vi "shape0.vi"() -> ()   [LabVIEW 2020]
uses:
  bee2abb7-c490-4ad6-bfc0-30ed72578e14.vi
panel:
  out "Array":cluster{"x":dbl, "y":dbl}[](array[cluster])
  in  "input variable":dbl=5.5 format="%#_13g"
  out "XY Graph":cluster{dbl[], dbl[]}(graph)
  # "e"
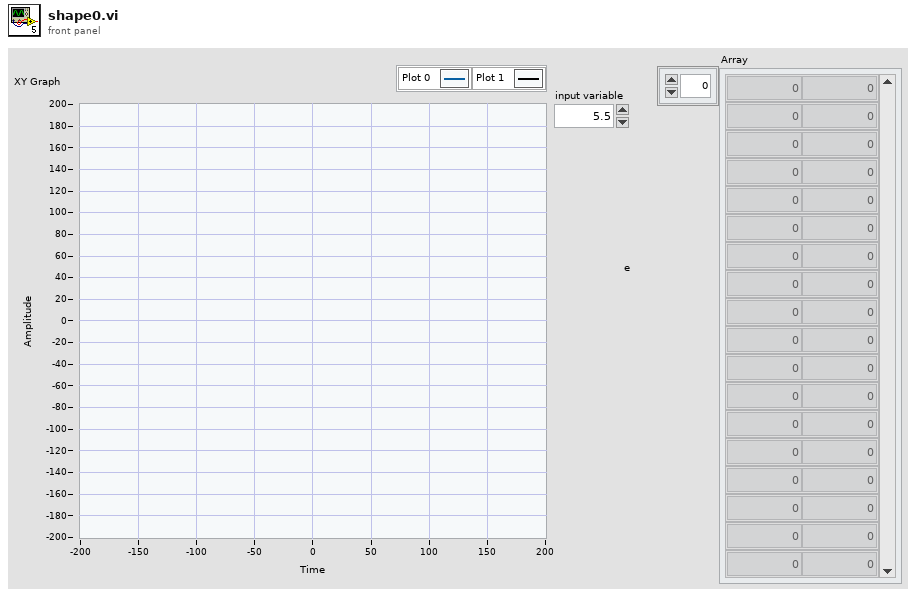
[diagram p1: front panel]
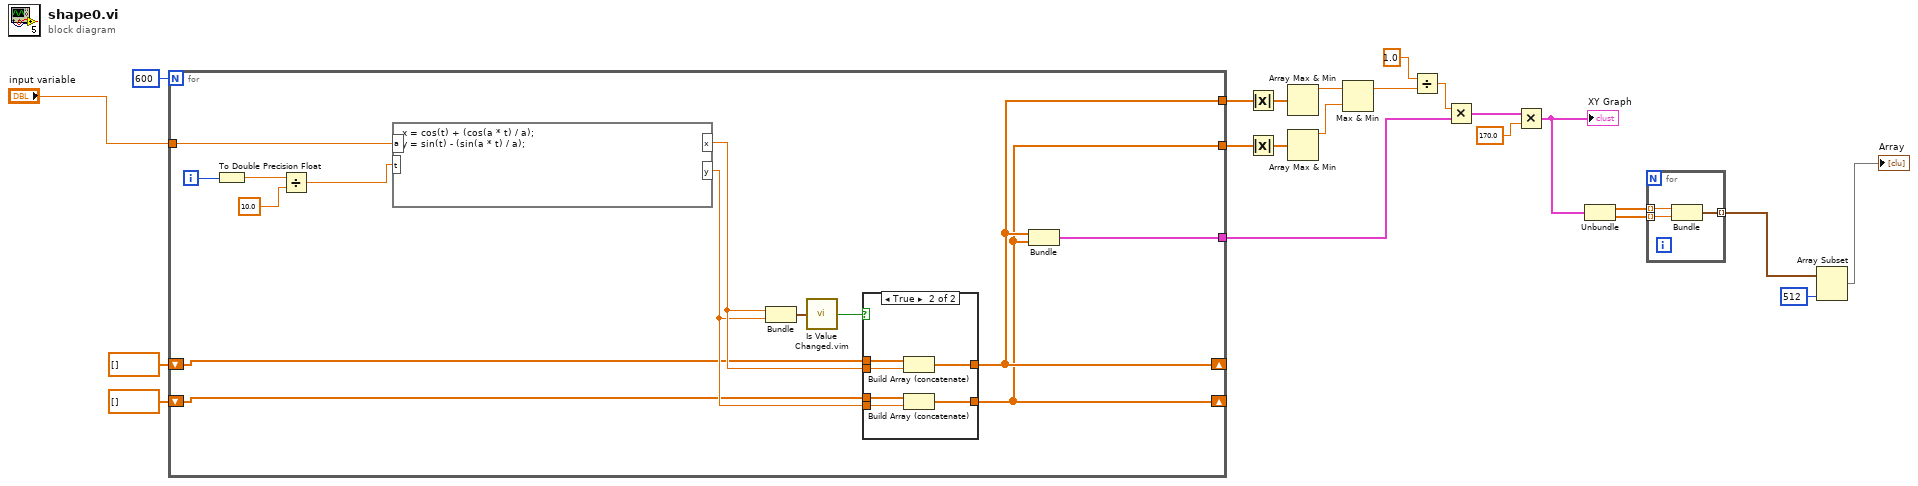
[diagram p0: block diagram]
diagram:
  n1 = for {
    N: 600 -> [_]
    tunnel: "input variable" -> [w36]
    shift-right: [w24] -> _
    shift-left: dbl[] [] -> [w31]
    shift-right: [w23] -> _
    shift-left: dbl[] [] -> [w30]
    tunnel: [w29] -> w9
    tunnel: [w24] -> w18
    tunnel: [w23] -> w17
    i -> [w28]
    n2 = To Double Precision Float(number=w28) -> (double precision float=w27:dbl)
    n3 = Divide(x=w27, y=10.0) -> (x/y=w25:dbl)
    n4 = formula code="x = cos(t) + (cos(a * t) / a);\ny = sin(t) - (sin(a * t) / a);"("a"=w36, "t"=w25) -> ("x"=w33:dbl, "y"=w32:dbl)
    n5 = Bundle("x"=w33, "y"=w32) -> (w35:cluster{"x":dbl, "y":dbl})  [unwired: 1 in]
    n6 = call "Is Value Changed.vim"("value"=w35) -> ("changed or first call?"=w34:bool)
    n7 = case shown="True" w34 {
      tunnel: w33 -> [_ w44]
      tunnel: w32 -> [_ w43]
      tunnel: [w38 w42] -> w24
      tunnel: [w37 w41] -> w23
      tunnel: w31 -> [w38 w40]
      tunnel: w30 -> [w37 w39]
      frame False {
      }
      frame True {
        n8 = Build Array (concatenate)(w40, w44) -> (w42:dbl[])
        n9 = Build Array (concatenate)(w39, w43) -> (w41:dbl[])
      }
    }
    n10 = Bundle(w24, w23) -> (w29:cluster{dbl[], dbl[]})  [unwired: 1 in]
  }
  n11 = Absolute Value(x=w18) -> (abs(x)=w16:dbl[])
  n12 = Absolute Value(x=w17) -> (abs(x)=w15:dbl[])
  n13 = Array Max & Min(array=w16) -> (max value=w14:dbl)  [unwired: 3 out]
  n14 = Array Max & Min(array=w15) -> (max value=w13:dbl)  [unwired: 3 out]
  n15 = Max & Min(x=w14, y=w13) -> (max(x,y)=w12:dbl)  [unwired: 1 out]
  n16 = Divide(x=1.0, y=w12) -> (x/y=w10:dbl)
  n17 = Multiply(x=w10, y=w9) -> (x*y=w8:cluster{dbl[], dbl[]})
  n18 = Multiply(x=w8, y=170.0 ("x")) -> (x*y=w6:cluster{dbl[], dbl[]})
  "XY Graph" <- w6
  n19 = Unbundle(w6) -> (w5:dbl[], w4:dbl[])
  n20 = for {
    tunnel: w5 -> [w47] mode=indexing
    tunnel: w4 -> [w46] mode=indexing
    tunnel: [w45] -> w3 mode=indexing
    n21 = Bundle("x"=w47, "y"=w46) -> (w45:cluster{"x":dbl, "y":dbl})  [unwired: 1 in]
  }
  n22 = Array Subset(array=w3, length=512) -> (→"Array":cluster{"x":dbl, "y":dbl}[])  [unwired: 1 in]
